vi "Get Boolean from Recipe.vi"(7 "Test Class in":refnum<class "Test Class.lvclass">, 8 "error in (no error)":errorcluster, 11 "Name":string) -> (0 "error out":errorcluster, 2 "found?":bool, 3 "Value":bool)   [LabVIEW 2017, in "Test Class.lvclass"]
uses:
  Test Class.lvclass
  Classes/Application/Class/Application.lvclass
  Classes/Test Recipe/Class/Test Recipe.lvclass
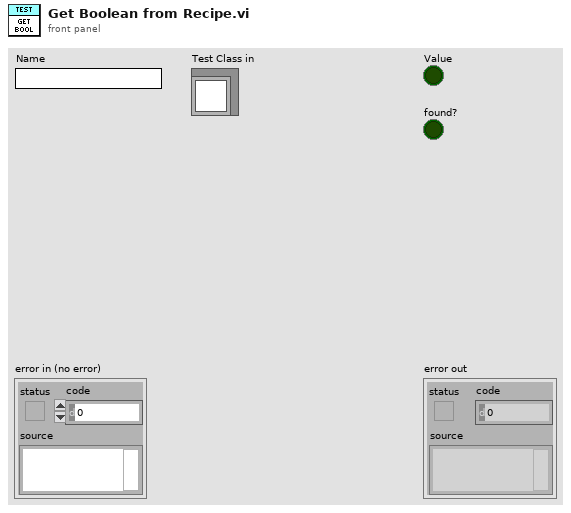
[diagram p1: front panel]
types:
  T1 = typedef "Application.lvlib/App Properties.lvclass/Class Properties -- Cluster.ctl" = cluster{"UUT Info":T2[], "Test Information":refnum<vi>, "Gold Board":refnum<class "Golden Board.lvclass">, "Test Recipe":refnum<class "Test Recipe.lvclass">, "Instruments":refnum<class "Instrument.lvclass">[], "Mode":T3, "Test Results":T4[], "Station Config":refnum<class "Station Config.lvclass">, "Variable Engine":refnum<class "Variable Engine.lvclass">}
  T2 = typedef "Application.lvlib/App Properties.lvclass/UUT Reference -- Cluster.ctl" = cluster{"Serial Number Reference":refnum<vi>, "Status Message Reference":refnum<vi>}
  T3 = typedef "Application.lvlib/Application.lvclass/Op Mode -- Enum.ctl" = u16
  T4 = typedef "Application.lvlib/App Properties.lvclass/Test Result -- Cluster.ctl" = cluster{"Position":i32, "Pass":bool, "Fail Codes":string}
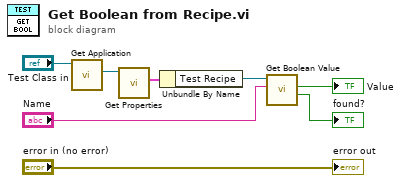
[diagram p0: block diagram]
diagram:
  n1 = call "Get Application.vi"("Test Class in"="Test Class in") -> ("Application.lvlib:Application.lvclass"=w7:refnum<class "Application.lvclass">)  [unwired: 9 in, 1 out]
  n2 = call "Get Properties.vi"("Acrobat Template in"=w7) -> ("Class Properties"=w6:T1)  [unwired: 8 in, 2 out]
  n3 = Unbundle By Name(w6) -> ("Test Recipe"=w4:refnum<class "Test Recipe.lvclass">)
  n4 = call "Get Boolean Value.vi"("Name"="Name", "Test Recipe in"=w4) -> ("found?"=→"found?":bool, "Value"=→"Value":bool)  [unwired: 6 in, 2 out]
  "error out" <- "error in (no error)"
